vi "DisplayArrayOfTimeStamps.vi"(3 "stop":bool, 4 "Array Of TimeStamps":timestamp[](array[timestamp])) -> (0 "Time Stamp 3":timestamp, 1 "Time Stamp 2":timestamp, 2 "Time Stamp":timestamp)   [LabVIEW 2011]
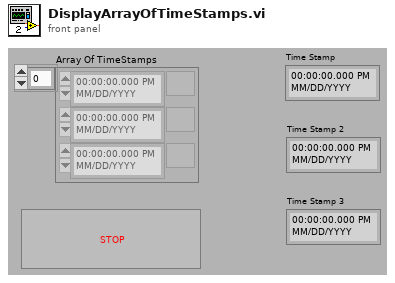
[diagram p1: front panel]
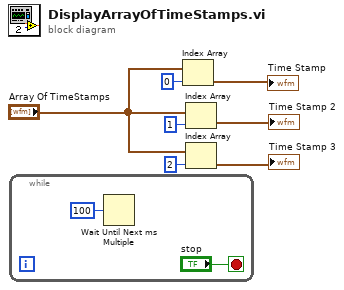
[diagram p0: block diagram]
diagram:
  n1 = while {
    stop <- "stop" stop-if-true
    n2 = Wait Until Next ms Multiple(millisecond multiple=u32 100) -> ()  [unwired: 1 out]
  }
  n3 = Index Array(array="Array Of TimeStamps", index=0) -> (element=→"Time Stamp":timestamp)
  n4 = Index Array(array="Array Of TimeStamps", index=1) -> (element=→"Time Stamp 2":timestamp)
  n5 = Index Array(array="Array Of TimeStamps", index=2) -> (element=→"Time Stamp 3":timestamp)
